vi "Configure AO Channel.vi"(7 "index":i32, 8 "error in":errorcluster, 10 "config":cluster{"carrier":dbl, "level":dbl}, 11 "host in":refnum<class "LIA Host Interface FPGA.lvclass">) -> (0 "error out":errorcluster, 3 "host out":refnum<class "LIA Host Interface FPGA.lvclass">)   [LabVIEW 2017, in "LIA Host Interface FPGA.lvclass"]
uses:
  LIA Host Interface FPGA.lvclass
  Properties/FpgaSession_GET.vi
  host/Lock-In Amplifier Example Host.lvlib
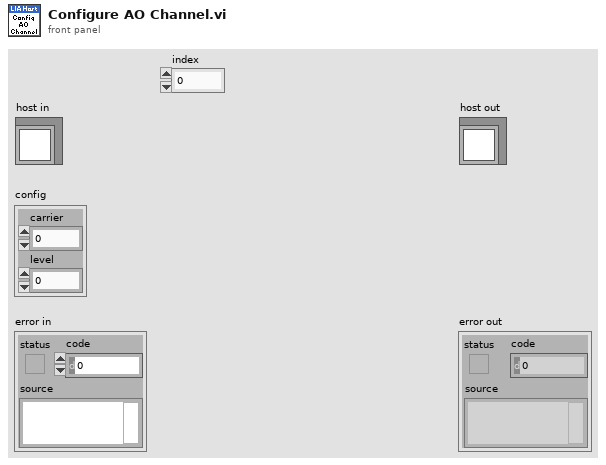
[diagram p1: front panel]
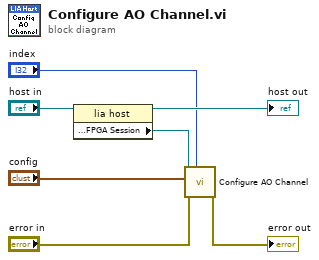
[diagram p0: block diagram]
diagram:
  n1 = property class="lia host"(reference="host in") -> (reference out=→"host out":refnum<class "LIA Host Interface FPGA.lvclass">, "Properties:FPGA Session"=w5:refnum<k20>)  [unwired: 1 in, 1 out]
  n2 = call "Configure AO Channel.vi"("index"="index", "error in"="error in", "config"="config", "fpga session in"=w5) -> ("error out"=→"error out":errorcluster)  [unwired: 6 in, 1 out]
